vi "Template Module.vi"(11 "Message Input":T1) -> (0 "error out":errorcluster, 5 "Message Output":T1)   [LabVIEW 2019]
uses:
  Channel Messages/Bundle Module Message/Bundle Module Message.xnode
  <extravilib>/ChannelInstances/Event Messenger-c(str,var).lvlib
  a9fd2b0d-eda1-479f-a41a-ee6a56868c0b.vi
  Template Module Cases.ctl
  5ed4f954-7074-48a6-b052-662a9e35750f.vi
  Last Ack.ctl
  Template Module Data.ctl
  <extravilib>/ChannelInstances/Event Messenger-c(str,var)/ChannelOp.ctl
  d0d43b5b-5edf-4743-83e5-19057c582713.vi
  <extravilib>/ChannelInstances/Event Messenger-c(str,var)/))Channel.ctl
panel:
  out "Log":string
  in  "module_interface":map{string, variant}(c390)={"Abort"=variant, "Handle Last Ack"=variant, "_Handle Error"=variant, "_Init"=variant}
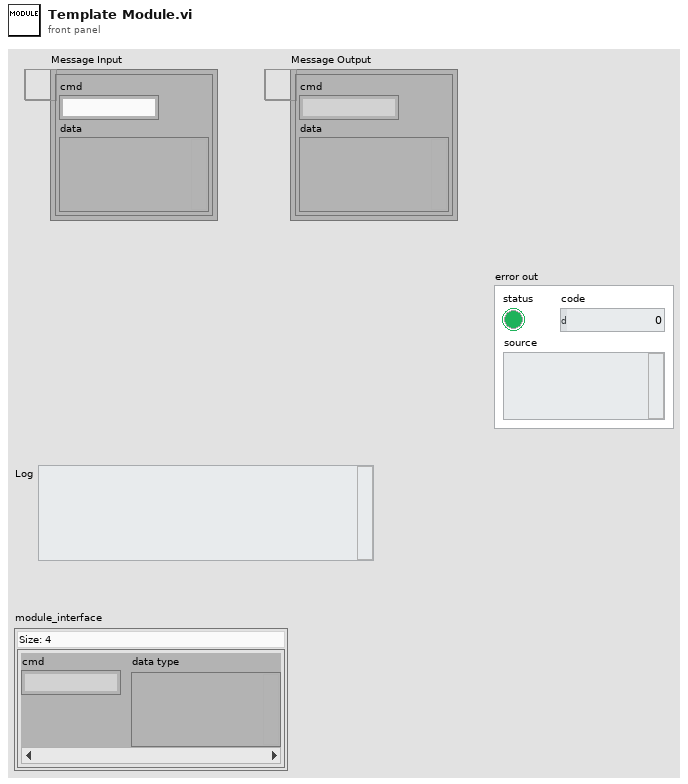
[diagram p1: front panel]
types:
  T1 = typedef "Event Messenger-c(str,var).lvlib/))Channel.ctl" = refnum<queue>
  T2 = typedef "Template Module Data.ctl" = cluster{"Ident":string, "Numeric":i32}
  T3 = typedef "Template Module Cases.ctl" = enum16{"Abort", "Handle Last Ack", "_Handle Error", "_Init"}
  T4 = typedef "Event Messenger-c(str,var).lvlib/ChannelOp.ctl" = enum16{"init", "write", "register", "replicate", "probe"}
  T5 = typedef "Last Ack.ctl" = cluster{"Ident":string, "Error Report":errorcluster, "State ":variant}
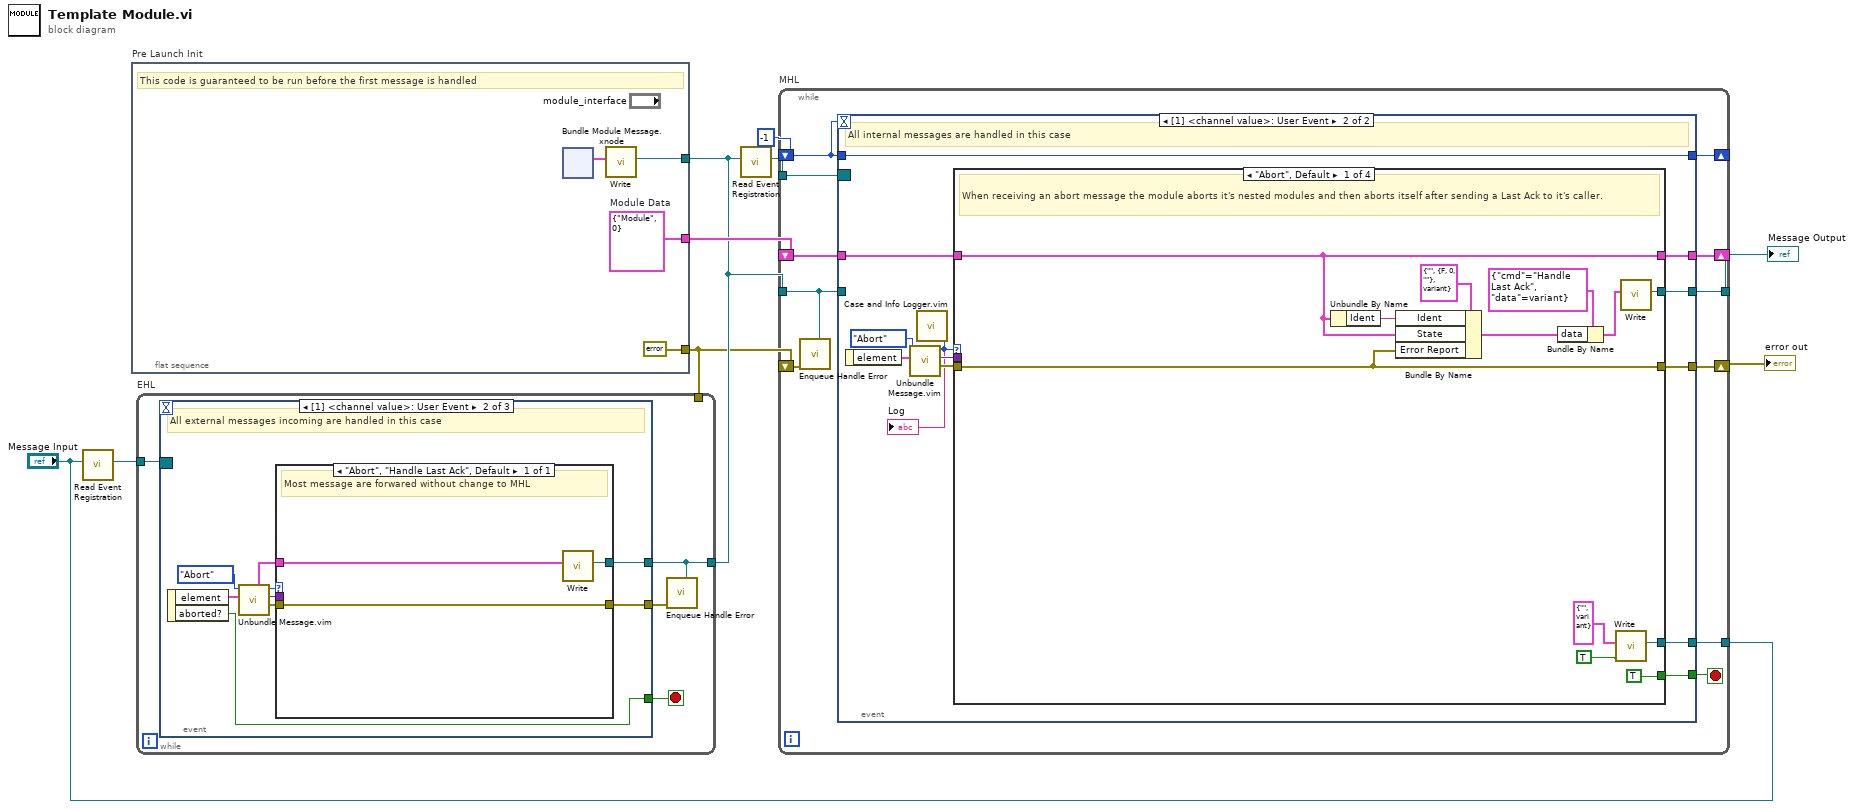
[diagram p0: block diagram]
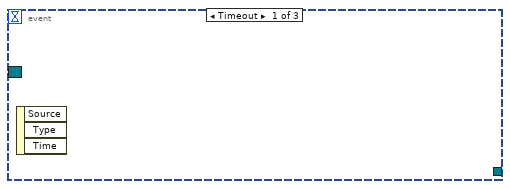
[diagram p2: hidden frame]
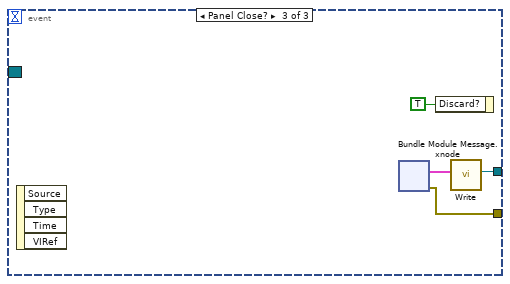
[diagram p3: hidden frame]
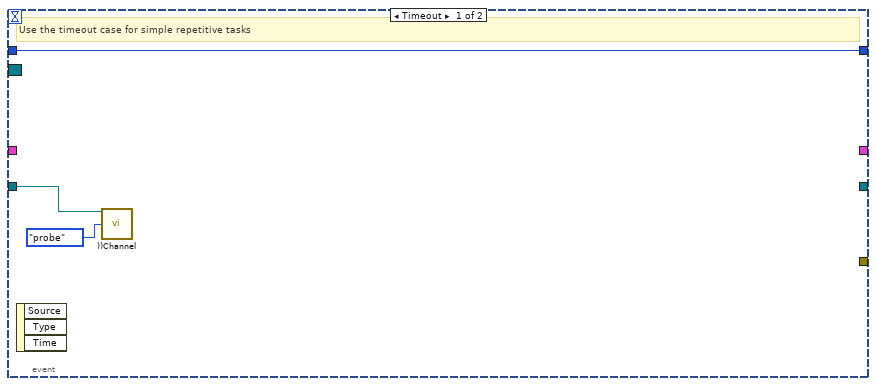
[diagram p4: hidden frame]
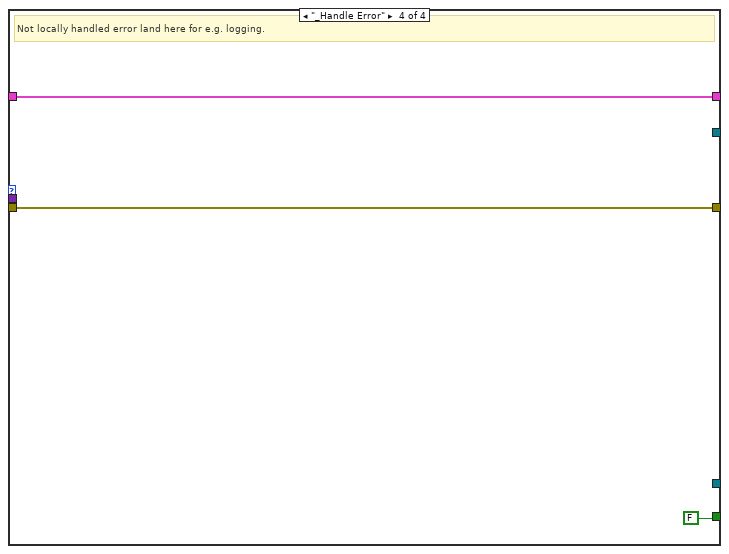
[diagram p7: hidden frame]
diagram:
  n1 = call <extravilib>:"Read Event Registration.vi"("channel"="Message Input") -> ("event registration refnum"=w6:refnum<event-registration>)  [unwired: 10 in]
  n2 = flat-sequence "Pre Launch Init" {
    tunnel: [w12] -> w4
    tunnel: [w11] -> w7
    tunnel: [errorcluster {"status"=FALSE, "code"=0, "source"=""} ("error IO")] -> w3
    frame #0 {
      w11 = T2 {"Ident"="Module", "Numeric"=0}  # Module Data
      # "This code is guaranteed to be run before the first message is handled"
      n3 = xnode "Bundle Module Message.xnode"() -> ("message"=w13:cluster{"cmd":string, "data":variant})  [unwired: 2 in, 1 out]
      n4 = call <extravilib>:"Write.vi"("element"=w13) -> ("channel"=w12:T1)  [unwired: 9 in, 1 out]
    }
  }
  n5 = while "EHL" {
    tunnel: w6 -> [w22]
    tunnel: w4 -> [w19]
    tunnel: w3 -> [_]
    stop <- w21 stop-if-true
    n6 = event shown="[1] <channel value>: User Event" {
      selector: w22 -> [_ _ _]
      dyn-events: _ -> [_ _ _]
      timeout: _ -> [_ _ _]
      tunnel: [_ w27 _] -> w21
      tunnel: [_ w25 w36] -> w19
      tunnel: [_ w24 w35] -> w20
      event Timeout {
        n7 = event-data() -> ()  [unwired: 1 in, 3 out]
      }
      event User Event {
        # "All external messages incoming are handled in this case"
        n8 = event-data() -> ("element"=w31:cluster{"cmd":string, "data":variant}, "aborted?"=w27:bool)  [unwired: 1 in]
        n9 = call "Unbundle Message.vim"("message"=w31, "case type"=Template_Module_Cases."Abort" ("Channeld Module Cases")) -> ("error out"=w23:errorcluster, "data"=w28:variant, "case"=w29:T3, "message dup"=w26:cluster{"cmd":string, "data":variant})  [unwired: 6 in]
        n10 = case shown="\"Abort\", \"Handle Last Ack\", Default" w29 {
          tunnel: w28 -> [_]
          tunnel: w26 -> [w33]
          tunnel: [w34] -> w25
          tunnel: [w32] -> w24
          tunnel: w23 -> [w32]
          frame "Abort", "Handle Last Ack", Default {
            # "Most message are forwared without change to MHL"
            n11 = call <extravilib>:"Write.vi"("element"=w33) -> ("channel"=w34:T1)  [unwired: 9 in, 1 out]
          }
        }
      }
      event Panel Close? {
        n12 = event-data() -> ()  [unwired: 1 in, 4 out]
        n13 = xnode "Bundle Module Message.xnode"() -> ("message"=w37:cluster{"cmd":string, "data":variant}, "error out"=w35:errorcluster)  [unwired: 2 in]
        n14 = event-data("Discard?"=TRUE) -> ()  [unwired: 1 in, 1 out]
        n15 = call <extravilib>:"Write.vi"("element"=w37) -> ("channel"=w36:T1)  [unwired: 9 in, 1 out]
      }
    }
    n16 = call "Enqueue Handle Error.vi"("MHL Channel in"=w19, "error in"=w20) -> ()  [unwired: 10 in]
  }
  n17 = call <extravilib>:"Read Event Registration.vi"("channel"=w4) -> ("event registration refnum"=w9:refnum<event-registration>)  [unwired: 10 in]
  n18 = while "MHL" {
    tunnel: w9 -> [w47]
    shift-right: [w53] -> _
    shift-left: -1 -> [w54]
    shift-right: [w51] -> _
    shift-left: w7 -> [w52]
    tunnel: [w50] -> w5
    shift-right: [w48] -> w2
    shift-left: w3 -> [w49]
    tunnel: w4 -> [w46]
    tunnel: "Message Input" -> [w44]
    stop <- w45 stop-if-true
    n19 = call "Enqueue Handle Error.vi"("MHL Channel in"=w46, "error in"=w49) -> ()  [unwired: 10 in]
    n20 = event shown="[1] <channel value>: User Event" {
      selector: w47 -> [_ _]
      dyn-events: _ -> [_ _]
      timeout: w54 -> [_ _]
      tunnel: w54 -> [w57 w70]
      tunnel: [w57 w70] -> w53
      tunnel: w52 -> [_ w68]
      tunnel: [_ w69] -> w51
      tunnel: [_ w64] -> w50
      tunnel: [_ w63] -> w48
      tunnel: w46 -> [w56 _]
      tunnel: [_ w62] -> w45
      tunnel: [_ w58] -> w44
      event Timeout {
        # "Use the timeout case for simple repetitive tasks"
        n21 = event-data() -> ()  [unwired: 1 in, 3 out]
        n22 = call <extravilib>:"))Channel.vi"("channel in"=w56, "channelOp"=ChannelOp."probe") -> ()  [unwired: 9 in, 5 out]
      }
      event User Event {
        # "All internal messages are handled in this case"
        n23 = event-data() -> ("element"=w67:cluster{"cmd":string, "data":variant})  [unwired: 1 in]
        n24 = call "Unbundle Message.vim"("message"=w67, "case type"=Template_Module_Cases."Abort" ("Channeld Module Cases")) -> ("error out"=w61:errorcluster, "data"=w66:variant, "case"=w60:T3)  [unwired: 6 in, 1 out]
        n25 = call "Case and Info Logger.vim"("Case"=w60) -> ("Log out"=→"Log":string)  [unwired: 10 in]
        n26 = case shown="\"Abort\", Default" w60 {
          tunnel: [w79 w84 w86 w89] -> w69
          tunnel: w68 -> [w79 w84 w86 w89]
          tunnel: w66 -> [_ _ _ _]
          tunnel: [w82 _ _ _] -> w64
          tunnel: w61 -> [w75 w83 w85 w88]
          tunnel: [w75 w83 w85 w88] -> w63
          tunnel: [TRUE _ _ FALSE] -> w62
          tunnel: [w73 _ _ _] -> w58
          frame "Abort", Default {
            # "When receiving an abort message the module aborts it's nested modules and then aborts itself after sending a Last Ack to it's caller."
            n27 = Unbundle By Name(w79) -> ("Ident"=w80:string)
            n28 = Bundle By Name(cluster=T5 {"Ident"="", "Error Report"={"status"=FALSE, "code"=0, "source"=""}, "State "=variant} ("Last Ack"), "Ident"=w80, "State"=w79, "Error Report"=w75) -> (w76:T5)
            n29 = Bundle By Name(cluster=cluster{"cmd":string, "data":variant} {"cmd"="Handle Last Ack", "data"=variant} ("message"), "data"=w76) -> (w77:cluster{"cmd":string, "data":variant})
            n30 = call <extravilib>:"Write.vi"("abort (F)"=TRUE, "element"=cluster{"cmd":string, "data":variant} {"cmd"="", "data"=variant}) -> ("channel"=w73:T1)  [unwired: 8 in, 1 out]
            n31 = call <extravilib>:"Write.vi"("element"=w77) -> ("channel"=w82:T1)  [unwired: 9 in, 1 out]
          }
          frame "_Init" {
          }
          frame "Handle Last Ack" {
            # "Last Ack is the message a nested module sends to it's caller when aborted."
          }
          frame "_Handle Error" {
            # "Not locally handled error land here for e.g. logging."
          }
        }
      }
    }
  }
  "Message Output" <- w5
  "error out" <- w2
